vi "Dialog Box 1 Button.vi"(0 "Font Name":string="Arial", 5 "Input":string caption="Message", 7 "OK Button":bool, 9 "Button Name (\"OK\")":string="OK", 11 "Font Size":u32=24, 12 "Font Color":u32) -> ()   [LabVIEW 2016]
doc: "This VI is similar to the One Button Dialog VI included with LabVIEW. The VI allows a user to customize the text in a dialog box. Customizable features include: font face, color, and size. The size and font customizations affect both message text and button text. A user may also customize the position at which the dialog box appears. This is accomplished by double clicking the icon, and then configuring the settings located by choosing File>>VI Properties>>Window Run-Time Position."
uses:
  controls/Dialog Message.ctl
panel:
  out "Display Message":T1 caption="Message"
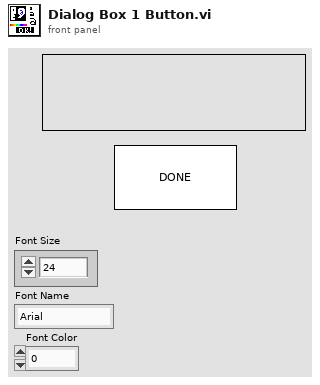
[diagram p1: front panel]
types:
  T1 = typedef "Dialog Message.ctl" = string
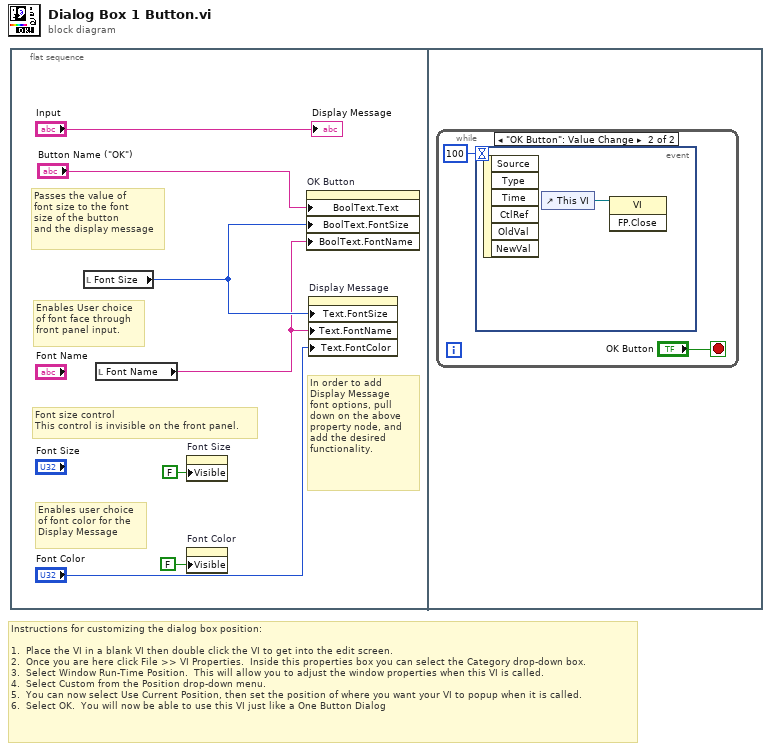
[diagram p0: block diagram]
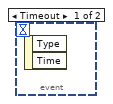
[diagram p2: hidden frame]
diagram:
  # "Instructions for customizing the dialog box position:\n\n1.  Place the VI in a blank VI then double click the VI to get into the edit screen.  \n2.  Once you are here click File >> VI Properties.  Inside this properties box you can select the Category drop-down box.\n3.  Select Window Run-Time Position.  This will allow you to adjust the window properties when this VI is called.\n4.  Select Custom from the Position drop-down menu.\n5.  You can now select Use Current Position, then set the position of where you want your VI to popup when it is called.\n6.  Select OK.  You will now be able to use this VI just like a One Button Dialog"
  n1 = flat-sequence {
    frame #0 {
      # "In order to add Display Message\nfont options, pull \ndown on the above property node, and add the desired functionality."
      # "Enables user choice\nof font color for the \nDisplay Message"
      # "Enables User choice\nof font face through\nfront panel input."
      # "Passes the value of \nfont size to the font\nsize of the button \nand the display message"
      # "Font size control \nThis control is invisible on the front panel."
      n2 = local read "Font Size"() -> (w5:u32)
      n3 = local read "Font Name"() -> (w3:string)
      n4 = property on="Font Size" class="DigNum (strict)"("Visible"=FALSE) -> ()  [unwired: 2 in, 2 out]
      n5 = property on="Font Color" class="DigNum (strict)"("Visible"=FALSE) -> ()  [unwired: 2 in, 2 out]
      n6 = property on="OK Button" class="Bool"("BoolText.Text"="Button Name (\"OK\")", "BoolText.FontSize"=w5, "BoolText.FontName"=w3) -> ()  [unwired: 2 in, 2 out]
      n7 = property on="Display Message" class="Str (strict)"("Text.FontSize"=w5, "Text.FontName"=w3, "Text.FontColor"="Font Color") -> ()  [unwired: 2 in, 2 out]
      "Display Message" <- "Input"
    }
    frame #1 {
      n8 = while {
        stop <- "OK Button" stop-if-true
        n9 = event shown="[1] \"OK Button\": Value Change" {
          selector: _ -> [_ _]
          dyn-events: _ -> [_ _]
          timeout: 100 -> [_ _]
          event Timeout {
            n10 = event-data() -> ()  [unwired: 3 out]
          }
          event "OK Button": Value Change {
            n11 = event-data() -> ()  [unwired: 7 out]
            n12 = control-ref of="This VI"() -> (w10:refnum<vi>)
            n13 = invoke class="VI" method="FP.Close"(reference=w10) -> ()  [unwired: 2 in, 3 out]
          }
        }
      }
    }
  }
